vi "路径查找创建-报警记录清单.vi"() -> (0 "累积剂量导出目录":path, 5 "调试选项路径":path, 8 "短信通知配置文件":path, 9 "蜂鸣音效文件路径":path, 10 "帮助文档路径":path, 11 "报表模板":path, 14 "配置文件":path, 15 "累积剂量配置文件":path, 16 "缓存数据文件夹":path, 17 "报警记录清单":path, 18 "数据库路径":path, 19 "报表文件夹":path)   [LabVIEW 2017]
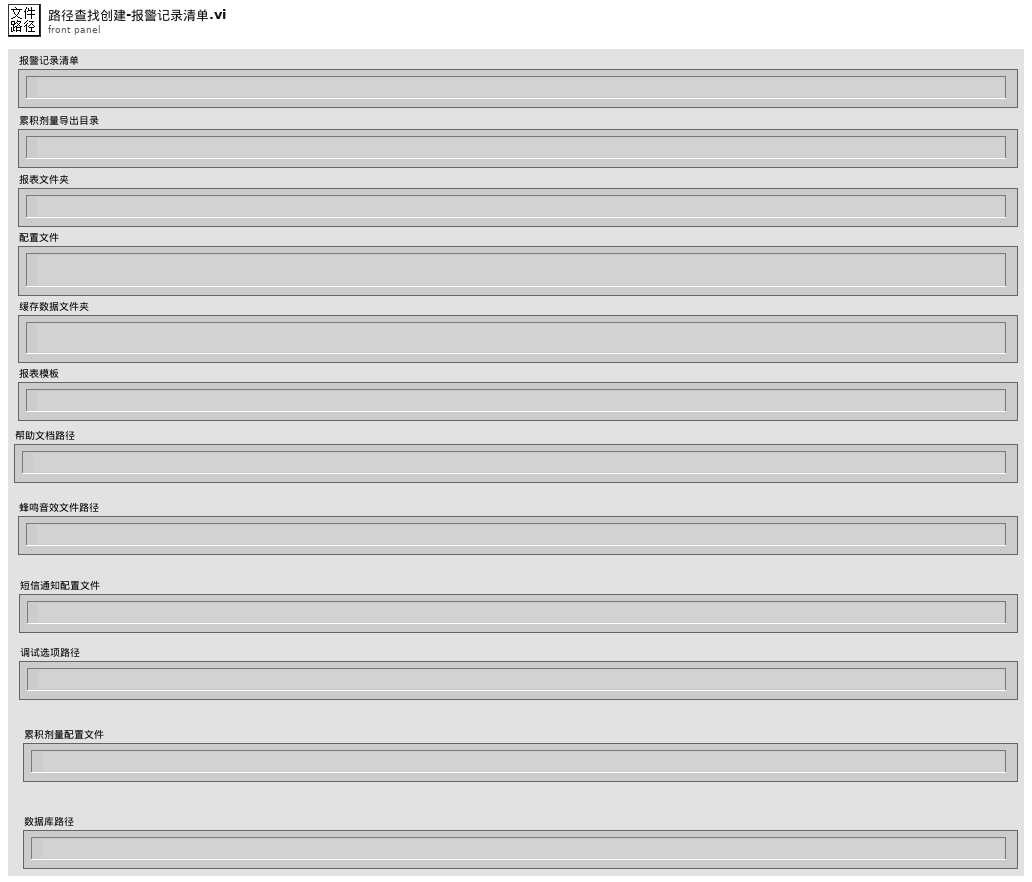
[diagram p1: front panel]
types:
  T1 = enum16{"open", "replace", "create", "open or create", "replace or create", "replace or create with confirmation"}
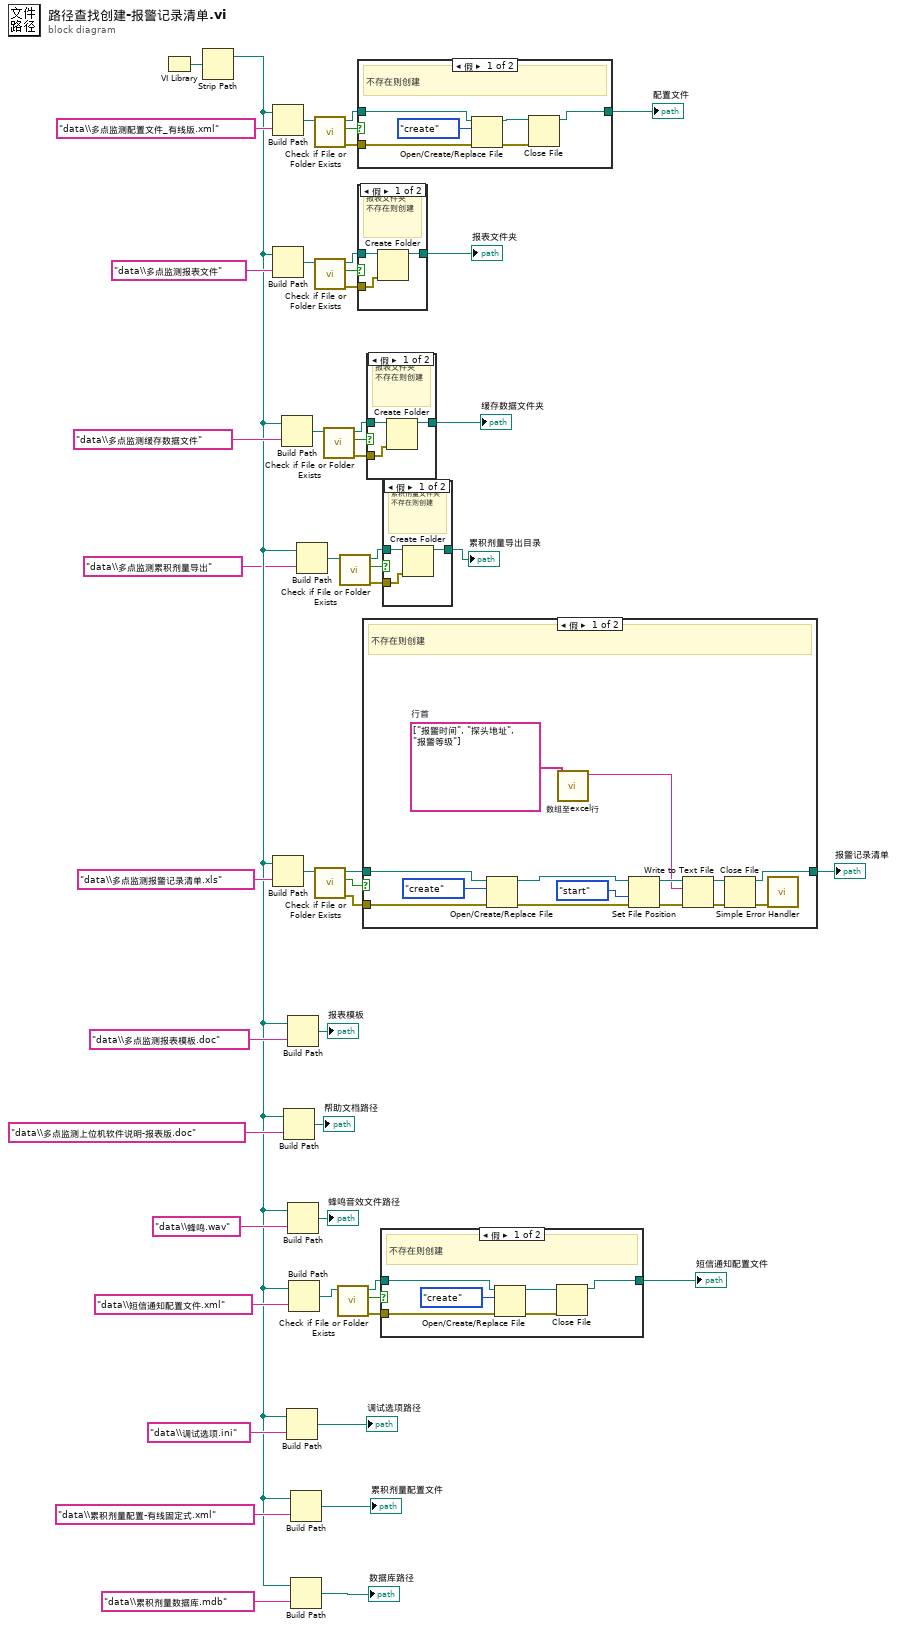
[diagram p0: block diagram]
diagram:
  n1 = VI Library() -> (path=w46:path)
  n2 = Strip Path(path=w46) -> (stripped path=w7:path)  [unwired: 1 out]
  n3 = Build Path(base path=w7, name or relative path="data\\多点监测配置文件_有线版.xml" ("读报警文件")) -> (appended path=w33:path)
  n4 = Build Path(base path=w7, name or relative path="data\\多点监测报表文件" ("读报警文件")) -> (appended path=w42:path)
  n5 = Build Path(base path=w7, name or relative path="data\\多点监测报警记录清单.xls" ("读报警文件")) -> (appended path=w49:path)
  n6 = Build Path(base path=w7, name or relative path="data\\多点监测缓存数据文件" ("读报警文件")) -> (appended path=w27:path)
  n7 = Build Path(base path=w7, name or relative path="data\\多点监测上位机软件说明-报表版.doc" ("读报警文件")) -> (appended path=→"帮助文档路径":path)
  n8 = Build Path(base path=w7, name or relative path="data\\调试选项.ini" ("读报警文件")) -> (appended path=→"调试选项路径":path)
  n9 = Build Path(base path=w7, name or relative path="data\\多点监测报表模板.doc" ("读报警文件")) -> (appended path=→"报表模板":path)
  n10 = Build Path(base path=w7, name or relative path="data\\蜂鸣.wav" ("读报警文件")) -> (appended path=→"蜂鸣音效文件路径":path)
  n11 = Build Path(base path=w7, name or relative path="data\\短信通知配置文件.xml" ("读报警文件")) -> (appended path=w15:path)
  n12 = Build Path(base path=w7, name or relative path="data\\累积剂量配置-有线固定式.xml" ("读报警文件")) -> (appended path=→"累积剂量配置文件":path)
  n13 = Build Path(base path=w7, name or relative path="data\\累积剂量数据库.mdb" ("读报警文件")) -> (appended path=→"数据库路径":path)
  n14 = Build Path(base path=w7, name or relative path="data\\多点监测累积剂量导出" ("读报警文件")) -> (appended path=w2:path)
  n15 = call <vilib>:"Check if File or Folder Exists.vi"("path"=w33) -> ("error out"=w34:errorcluster, "file or folder exists?"=w36:bool, "dup path"=w35:path)  [unwired: 8 in]
  n16 = call <vilib>:"Check if File or Folder Exists.vi"("path"=w42) -> ("error out"=w39:errorcluster, "file or folder exists?"=w41:bool, "dup path"=w40:path)  [unwired: 8 in]
  n17 = call <vilib>:"Check if File or Folder Exists.vi"("path"=w49) -> ("error out"=w48:errorcluster, "file or folder exists?"=w45:bool, "dup path"=w47:path)  [unwired: 8 in]
  n18 = call <vilib>:"Check if File or Folder Exists.vi"("path"=w27) -> ("error out"=w30:errorcluster, "file or folder exists?"=w28:bool, "dup path"=w29:path)  [unwired: 8 in]
  n19 = call <vilib>:"Check if File or Folder Exists.vi"("path"=w15) -> ("error out"=w16:errorcluster, "file or folder exists?"=w18:bool, "dup path"=w17:path)  [unwired: 8 in]
  n20 = call <vilib>:"Check if File or Folder Exists.vi"("path"=w2) -> ("error out"=w3:errorcluster, "file or folder exists?"=w5:bool, "dup path"=w4:path)  [unwired: 8 in]
  n21 = case shown="假" w36 {
    tunnel: w34 -> [w55 _]
    tunnel: w35 -> [w54 w57]
    tunnel: [w51 w57] -> w37
    frame False {
      # "不存在则创建"
      n22 = Open/Create/Replace File(file path (use dialog)=w54, error in=w55, operation (0:open)=T1."create" ("操作(0:open)")) -> (refnum out=w53:refnum<file>, error out=w52:errorcluster)  [unwired: 3 in, 1 out]
      n23 = Close File(refnum=w53, error in=w52) -> (path=w51:path)  [unwired: 1 out]
    }
    frame True {
      # "存在则输出"
    }
  }
  "配置文件" <- w37
  n24 = case shown="假" w41 {
    tunnel: w40 -> [w60 w61]
    tunnel: w39 -> [w59 _]
    tunnel: [w58 w61] -> w38
    frame False {
      # "报表文件夹\n不存在则创建"
      n25 = Create Folder(path (use dialog)=w60, error in=w59) -> (created path=w58:path)  [unwired: 1 in, 2 out]
    }
    frame True {
    }
  }
  "报表文件夹" <- w38
  n26 = case shown="假" w45 {
    tunnel: w48 -> [w74 _]
    tunnel: w47 -> [w73 w76]
    tunnel: [w64 w76] -> w44
    frame False {
      w63 = string[] ["报警时间", "探头地址", "报警等级"]  # 行首
      # "不存在则创建"
      n27 = Open/Create/Replace File(file path (use dialog)=w73, error in=w74, operation (0:open)=T1."create" ("操作(0:open)")) -> (refnum out=w66:refnum<file>, error out=w65:errorcluster)  [unwired: 3 in, 1 out]
      n28 = call "数组至excel行.vi"("数组"=w63) -> ("字符串"=w62:string)  [unwired: 10 in]
      n29 = Set File Position(refnum=w66, from (0:start)=enum16{"start", "end", "current"}."start" ("自（0:起始）"), error in=w65) -> (refnum out=w69:refnum<file>, error out=w68:errorcluster)  [unwired: 1 out]
      n30 = Write to Text File(file (use dialog)=w69, text=w62, error in=w68) -> (refnum out=w71:refnum<file>, error out=w72:errorcluster)  [unwired: 2 out]
      n31 = Close File(refnum=w71, error in=w72) -> (path=w64:path, error out=w70:errorcluster)
      n32 = call <vilib>:"Simple Error Handler.vi"("error in (no error)"=w70) -> ()  [unwired: 1 in, 8 out]
    }
    frame True {
      # "存在则输出"
    }
  }
  "报警记录清单" <- w44
  n33 = case shown="假" w28 {
    tunnel: w29 -> [w79 w80]
    tunnel: w30 -> [w78 _]
    tunnel: [w77 w80] -> w31
    frame False {
      # "报表文件夹\n不存在则创建"
      n34 = Create Folder(path (use dialog)=w79, error in=w78) -> (created path=w77:path)  [unwired: 1 in, 2 out]
    }
    frame True {
    }
  }
  "缓存数据文件夹" <- w31
  n35 = case shown="假" w18 {
    tunnel: w16 -> [w85 _]
    tunnel: w17 -> [w84 w87]
    tunnel: [w81 w87] -> w14
    frame False {
      # "不存在则创建"
      n36 = Open/Create/Replace File(file path (use dialog)=w84, error in=w85, operation (0:open)=T1."create" ("操作(0:open)")) -> (refnum out=w83:refnum<file>, error out=w82:errorcluster)  [unwired: 3 in, 1 out]
      n37 = Close File(refnum=w83, error in=w82) -> (path=w81:path)  [unwired: 1 out]
    }
    frame True {
      # "存在则输出"
    }
  }
  "短信通知配置文件" <- w14
  n38 = case shown="假" w5 {
    tunnel: w4 -> [w90 w91]
    tunnel: w3 -> [w89 _]
    tunnel: [w88 w91] -> w1
    frame False {
      # "累积剂量文件夹\n不存在则创建"
      n39 = Create Folder(path (use dialog)=w90, error in=w89) -> (created path=w88:path)  [unwired: 1 in, 2 out]
    }
    frame True {
    }
  }
  "累积剂量导出目录" <- w1
